vi "LEDs_OFF.vi"(8 "error in (no error)":errorcluster, 11 "channel":refnum<k24>) -> (0 "error out":errorcluster)   [LabVIEW 2021]
uses:
  F:/2PhotonVision/psychometric_function_v2/lib/Grpc.Core.dll
  lib/Grpc.Core.dll
  F:/2PhotonVision/psychometric_function_v2/lib/FossilProtosSharp.dll
  lib/FossilProtosSharp.dll
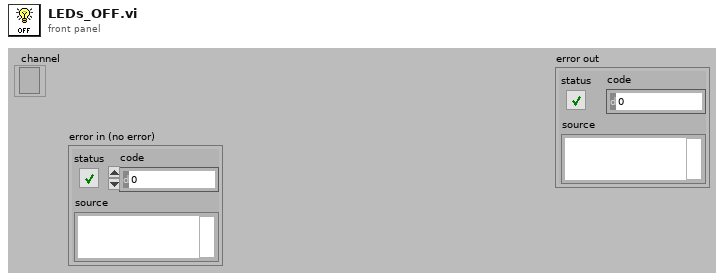
[diagram p1: front panel]
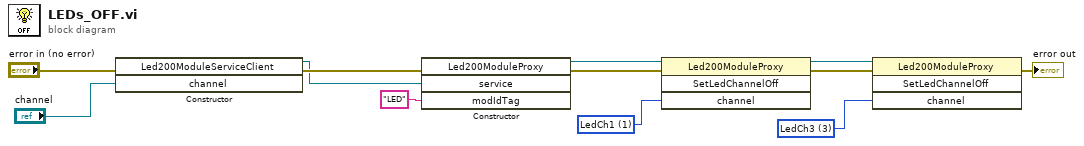
[diagram p0: block diagram]
diagram:
  w12 = 3 items=["LedChUnspecified", "LedCh1", "LedCh2", "LedCh3", "LedCh4"] ("channel")
  w10 = 1 items=["LedChUnspecified", "LedCh1", "LedCh2", "LedCh3", "LedCh4"] ("channel")
  n1 = constructor class="Led200ModuleServiceClient"(error in="error in (no error)", "channel"="channel") -> (reference out=w1:refnum<k24>, error out=w3:errorcluster)  [unwired: 2 in, 2 out]
  n2 = constructor class="Led200ModuleProxy"(error in=w3, "service"=w1, "modIdTag"="LED") -> (reference out=w5:refnum<k24>, error out=w6:errorcluster)  [unwired: 2 in, 3 out]
  n3 = invoke class="Led200ModuleProxy" method="SetLedChannelOff"(reference=w5, error in=w6, "channel"=w10) -> (reference out=w9:refnum<k24>, error out=w11:errorcluster)  [unwired: 1 in, 2 out]
  n4 = invoke class="Led200ModuleProxy" method="SetLedChannelOff"(reference=w9, error in=w11, "channel"=w12) -> (error out=→"error out":errorcluster)  [unwired: 1 in, 3 out]
